vi "GetRxWfmPath.vi"(11 "AllRxWfmName":string="aa.tdms,bb.tdms,dd.tdms") -> (3 "RxWfmNameArray":string[](array[string]))   [LabVIEW 2012]
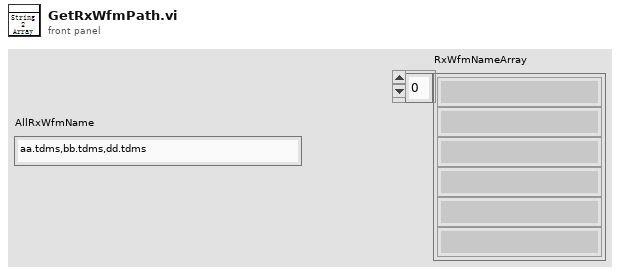
[diagram p1: front panel]
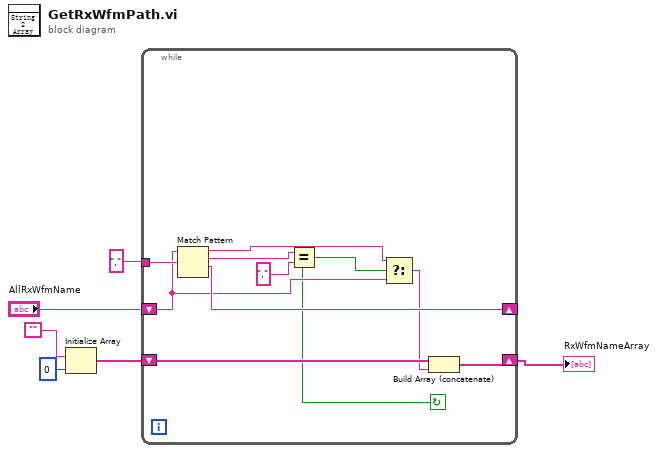
[diagram p0: block diagram]
diagram:
  n1 = Initialize Array("", 0 ("dimension size")) -> (w2:string[])
  n2 = while {
    tunnel: "," ("search string/char (-)") -> [w16]
    shift-right: [w13] -> _
    shift-left: "AllRxWfmName" -> [w10]
    shift-right: [w11] -> w1
    shift-left: w2 -> [w12]
    stop <- w7 continue-if-true
    n3 = Match Pattern(string=w10, regular expression=w16) -> (before substring=w9:string, match substring=w15:string, after substring=w13:string)  [unwired: 1 in, 1 out]
    n4 = Equal?(x=w15, y="," ("search string/char (-)")) -> (x = y?=w7:bool)
    n5 = Select(t=w9, s=w7, f=w10) -> (s? t:f=w8:string)
    n6 = Build Array (concatenate)(w12, w8) -> (w11:string[])
  }
  "RxWfmNameArray" <- w1
